vi "subvi-dll.vi"(4 "Numeric":dbl, 5 "Kernel":dbl[][](array[numeric]), 6 "Value":u8, 7 "bottom":i16, 8 "Real Matrix":T1, 9 "Real Matrix 2":T1, 10 "Real Matrix 3":T1, 11 "right":i16) -> (1 "image_data":dbl[][](array[numeric]), 2 "image_data 2":dbl[][](array[numeric]), 3 "image_data 3":dbl[][](array[numeric]))   [LabVIEW 2016]
uses:
  <vilib>/Analysis/Matrix/Datatypes/RealMatrix.ctl
  <vilib>/Analysis/Matrix/Numeric/Conversions/Matrix To Array - RM.vi
  <vilib>/Analysis/Matrix/NI_Matrix.lvlib
  ProcessingDLL4/x64/Debug/ProcessingDLL4.dll
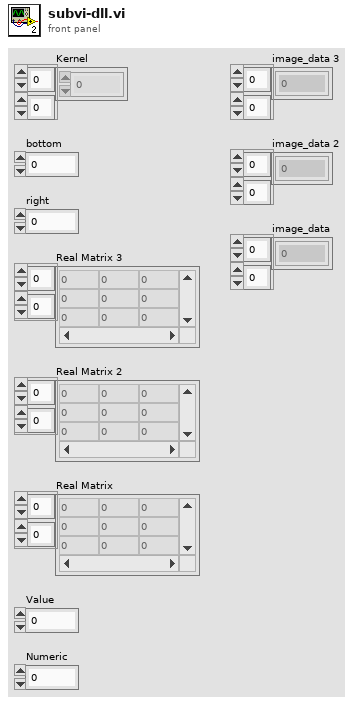
[diagram p1: front panel]
types:
  T1 = typedef "NI_Matrix.lvlib/RealMatrix.ctl" = dbl[][]
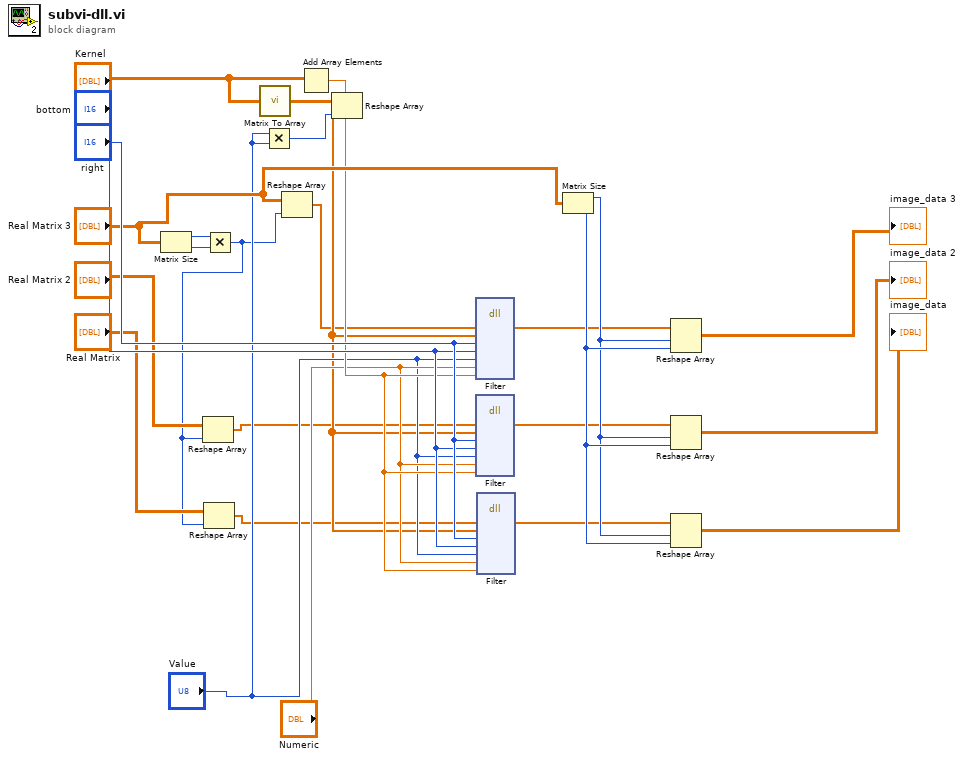
[diagram p0: block diagram]
diagram:
  n1 = Matrix Size(0:"Real Matrix 3") -> (1:w3:i32, 2:w4:i32)
  n2 = Multiply(x=w3, y=w4) -> (x*y=w11:i32)
  n3 = Reshape Array("Real Matrix 2", w11) -> (w12:dbl[])
  n4 = Reshape Array("Real Matrix", w11) -> (w13:dbl[])
  n5 = call-poly <vilib>:"Matrix To Array.vi"("Real Matrix"="Kernel") -> ("Real 2D Array"=w1:dbl[][])
  n6 = Multiply(x="Value", y="Value") -> (x*y=w2:u8)
  n7 = Reshape Array("Real Matrix 3", w11) -> (w5:dbl[])
  n8 = Add Array Elements(numeric array="Kernel") -> (sum=w17:dbl)
  n9 = Reshape Array(w1, w2) -> (w14:dbl[])
  n10 = dll-call lib="H:/11 sem/ProcessingDLL4/x64/Debug/ProcessingDLL4.dll" fn="Filter"("image_data"=w5, "image_kernel"=w14, "rows"="right", "columns"="bottom", "kernel_dim"="Value", "kernel_div"="Numeric", "div"=w17) -> ("image_data"=w6:dbl[])  [unwired: 10 in, 2 out]
  n11 = dll-call lib="H:/11 sem/ProcessingDLL4/x64/Debug/ProcessingDLL4.dll" fn="Filter"("image_data"=w12, "image_kernel"=w14, "rows"="right", "columns"="bottom", "kernel_dim"="Value", "kernel_div"="Numeric", "div"=w17) -> ("image_data"=w8:dbl[])  [unwired: 10 in, 2 out]
  n12 = dll-call lib="H:/11 sem/ProcessingDLL4/x64/Debug/ProcessingDLL4.dll" fn="Filter"("image_data"=w13, "image_kernel"=w14, "rows"="right", "columns"="bottom", "kernel_dim"="Value", "kernel_div"="Numeric", "div"=w17) -> ("image_data"=w7:dbl[])  [unwired: 10 in, 2 out]
  n13 = Matrix Size(0:"Real Matrix 3") -> (1:w9:i32, 2:w10:i32)
  n14 = Reshape Array(w6, w9, w10) -> (→"image_data 3":dbl[][])
  n15 = Reshape Array(w8, w9, w10) -> (→"image_data 2":dbl[][])
  n16 = Reshape Array(w7, w9, w10) -> (→"image_data":dbl[][])
